vi "test 01.vi"() -> ()   [LabVIEW 2020]
uses:
  UI_Actor/UI_Actor/UI_Actor.lvclass
  support/Actor Framework.lvlibp/Stop Msg/Stop Msg.lvclass
panel:
  out "PASS":bool
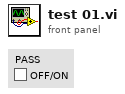
[diagram p1: front panel]
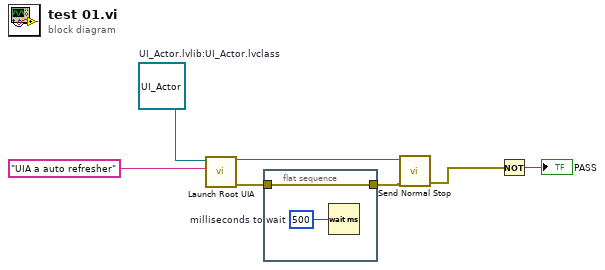
[diagram p0: block diagram]
diagram:
  w3 = refnum<class "UI_Actor.lvclass"> refnum  # UI_Actor.lvlib:UI_Actor.lvclass
  n1 = call "Launch Root UIA.vi"("Actor Name"="UIA a auto refresher", "UI_Actor in"=w3) -> ("error out"=w1:errorcluster, "Actor's Enqueuer"=w6:refnum<class "Message Enqueuer.lvclass">)  [unwired: 8 in]
  n2 = flat-sequence {
    tunnel: [w8] -> w2
    tunnel: w1 -> [w8]
    frame #0 {
      w9 = u32 500  # milliseconds to wait
      n3 = Wait (ms)(milliseconds to wait=w9) -> ()  [unwired: 1 out]
    }
  }
  n4 = call "Send Normal Stop.vi"("error in (no error)"=w2, "Message Enqueuer"=w6) -> ("error out"=w5:errorcluster)  [unwired: 9 in]
  n5 = Not(x=w5) -> (.not. x?=→"PASS":bool)
